vi "Uninstall startup application.vi"(8 "error in (no error)":errorcluster, 11 "RT Management in":refnum<class "RT Management.lvclass">) -> (0 "error out":errorcluster, 3 "RT Management out":refnum<class "RT Management.lvclass">)   [LabVIEW 2016, in "RT Management.lvlib" / "RT Management.lvclass"]
doc: "Uninstalls the startup application by deleting all contents inside the startup application folder and resetting the ni-rt.ini \"RTTarget.ApplicationPath\" key to \"startup.rtexe\". This VI does not restart the target."
uses:
  RT Management.lvclass
  controls/INI key.ctl
  File Transfer Behavior/File Transfer Behavior.lvclass
  RT Management.lvlib
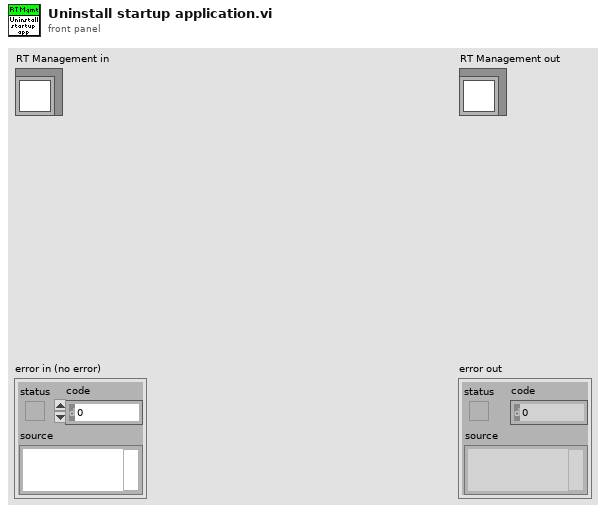
[diagram p1: front panel]
types:
  T1 = typedef "RT Management.lvlib/INI key.ctl" = cluster{"Section":string, "Key name":string, "Key value":string}
  T2 = typedef "RT Management.lvlib/RT Management.lvclass/Operating system.ctl" = enum16{"Unknown", "VxWorks", "PharLap", "Linux-ARM", "Linux-x64"}
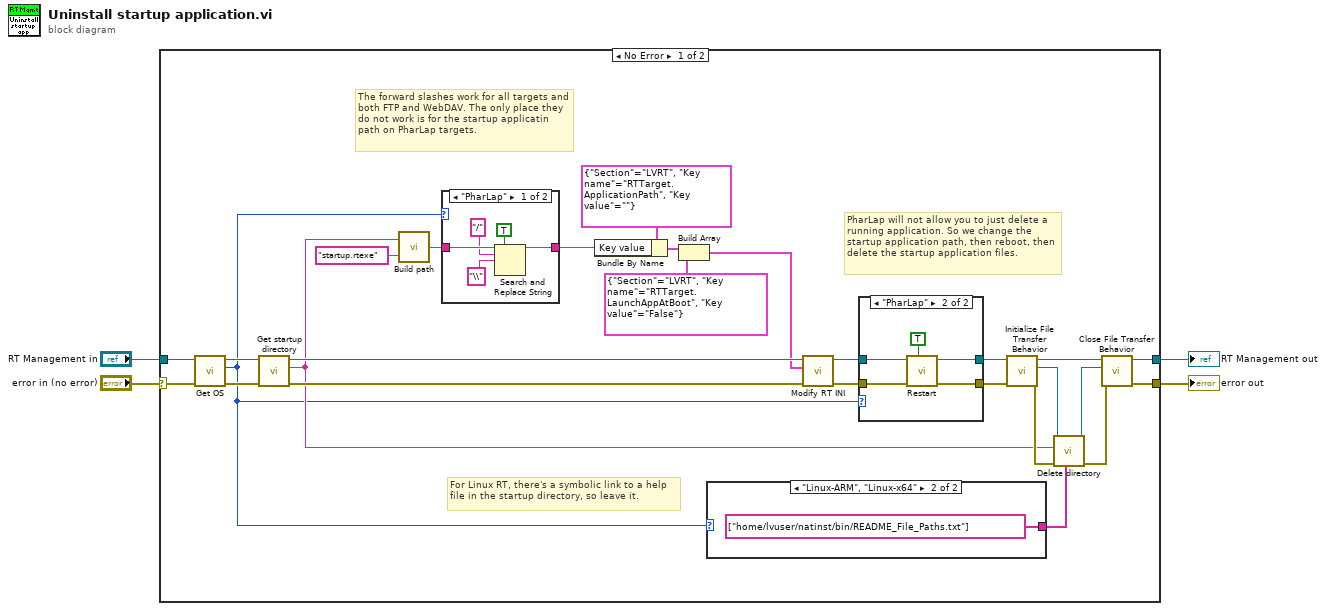
[diagram p0: block diagram]
diagram:
  n1 = case shown="No Error" "error in (no error)" {
    selector: "error in (no error)" -> [w26 w47]
    tunnel: [w6 w47] -> w3
    tunnel: [w7 w46] -> w1
    tunnel: "RT Management in" -> [w25 w46]
    frame No Error {
      # "For Linux RT, there's a symbolic link to a help file in the startup directory, so leave it."
      # "PharLap will not allow you to just delete a running application. So we change the startup application path, then reboot, then delete the startup application files."
      # "The forward slashes work for all targets and both FTP and WebDAV. The only place they do not work is for the startup applicatin path on PharLap targets."
      n2 = call "Get OS.vi"("error in (no error)"=w26, "RT Management in"=w25) -> ("error out"=w24:errorcluster, "Operating System"=w5:T2, "RT Management out"=w23:refnum<class "RT Management.lvclass">)  [unwired: 6 in, 1 out]
      n3 = call "Get startup directory.vi"("error in (no error)"=w24, "RT Management in"=w23) -> ("error out"=w16:errorcluster, "Startup directory"=w10:string, "RT Management out"=w17:refnum<class "RT Management.lvclass">)  [unwired: 7 in]
      n4 = call "Build path.vi"("Relative path"="startup.rtexe" ("Key value"), "Base path"=w10) -> ("Resulting path"=w9:string)
      n5 = case shown="\"PharLap\"" w5 {
        tunnel: w9 -> [w43 w44]
        tunnel: [w39 w44] -> w8
        frame "PharLap" {
          n6 = Search and Replace String(replace all?=TRUE ("replace all? (F)"), input string=w43, search string="/", replace string="\\" ("replace string (\"\")")) -> (result string=w39:string)  [unwired: 4 in, 3 out]
        }
        frame Default {
        }
      }
      n7 = Bundle By Name(cluster=T1 {"Section"="LVRT", "Key name"="RTTarget.ApplicationPath", "Key value"=""} ("INI_Key"), "Key value"=w8) -> (w18:T1)
      n8 = Build Array(w18, T1 {"Section"="LVRT", "Key name"="RTTarget.LaunchAppAtBoot", "Key value"="False"} ("INI_Key")) -> (w13:T1[])
      n9 = case shown="\"Linux-ARM\", \"Linux-x64\"" w5 {
        tunnel: [_ string[] ["home/lvuser/natinst/bin/README_File_Paths.txt"]] -> w22
        frame Default {
        }
        frame "Linux-ARM", "Linux-x64" {
        }
      }
      n10 = call "Modify RT INI.vi"("error in (no error)"=w16, "Keys to edit"=w13, "RT Management in"=w17) -> ("error out"=w15:errorcluster, "RT Management out"=w14:refnum<class "RT Management.lvclass">)  [unwired: 7 in]
      n11 = case shown="\"PharLap\"" w5 {
        tunnel: w15 -> [w32 w38]
        tunnel: w14 -> [w33 w37]
        tunnel: [w32 w35] -> w12
        tunnel: [w33 w34] -> w11
        frame Default {
        }
        frame "PharLap" {
          n12 = call "Restart.vi"("Wait until complete (true)"=TRUE, "error in (no error)"=w38, "RT Management in"=w37) -> ("error out"=w35:errorcluster, "RT Management out"=w34:refnum<class "RT Management.lvclass">)  [unwired: 6 in]
        }
      }
      n13 = call "Initialize File Transfer Behavior.vi"("error in (no error)"=w12, "RT Management in"=w11) -> ("error out"=w30:errorcluster, "File Transfer Behavior out"=w31:refnum<class "File Transfer Behavior.lvclass">, "RT Management out"=w29:refnum<class "RT Management.lvclass">)  [unwired: 7 in]
      n14 = call "Delete directory.vi"("Paths to exclude"=w22, "error in (no error)"=w30, "Directory"=w10, "File Transfer Behavior in"=w31) -> ("error out"=w28:errorcluster, "File Transfer Behavior out"=w27:refnum<class "File Transfer Behavior.lvclass">)  [unwired: 6 in]
      n15 = call "Close File Transfer Behavior.vi"("error in (no error)"=w28, "File Transfer Behavior in"=w27, "RT Management in"=w29) -> ("error out"=w6:errorcluster, "RT Management out"=w7:refnum<class "RT Management.lvclass">)  [unwired: 7 in]
    }
    frame Error {
    }
  }
  "error out" <- w3
  "RT Management out" <- w1
